vi "Camera_Crop_Setup.vi"(11 "value":T1={"L16 Linear Actuator"="", "XE 1000 Pump"="", "Camera1"="", "Camera2"="", "Img_Capt"=FALSE, "Actuator"=FALSE, "Pump"=FALSE, "Cam 1"=FALSE, "Cam 2"=FALSE, "Empty_Refill"=FALSE, "Crop"=FALSE, "Light intensity"=100, "Exposure Time"=1000.0, "Sample Name"="Test Sample", "Operator"="MRJ", "Calibration 1"=path "C:/Users/au540322/Desktop/IHS_Project/images/Debris/Debris_0/Debris_0_2019_06_01-23-32-49-686.PNG", "Calibration 2"=path "C:/Users/au540322/Desktop/IHS_Project/images/Debris/Debris_0/Debris_0_2019_06_01-23-32-49-686.PNG", "Framerate"=100, "Timeout Sample"=200, "Collection date"="", "Sample size threshold"=500, "Empty start"=1, "Command"="", "Station"="", "Species Name"="", "Other Notes"="", "Aperture"=enum."Item 0", "Image Process Queue Size"=500, "Image Save Queue Size"=500, "Overload threshold"=500, "Max Framerate"=100, "Rectangle 1"={"Left"=0, "Top"=0, "Right"=0, "Bottom"=0, "Rotation"=0.0}, "Rectangle 2"={"Left"=0, "Top"=0, "Right"=0, "Bottom"=0, "Rotation"=0.0}, "Detection Region %"=0.0, "Detect 1"=path "C:/Users/au540322/Desktop/IHS_Project/images/Debris/Debris_0/Debris_0_2019_06_01-23-32-49-686.PNG", "Detect 2"=path "C:/Users/au540322/Desktop/IHS_Project/images/Debris/Debris_0/Debris_0_2019_06_01-23-32-49-686.PNG", "Max large object threshold"=0, "Open(T)/Close(F)"=FALSE, "Img_Capt Begin"=FALSE, "Dispense Speed"=100, "Flush Size"=100, "Location"="Station", "Latitude"="Station", "Longitude"="Station", "Determiner"="Station", "Sex"="Station", "Camera1_Img"=refnum, "Camera2_Img"=refnum, "Img1_Orig_Disp"=refnum, "Img2_Orig_Disp"=refnum, "Img1_Orig_RGB"=refnum, "Img2_Orig_RGB"=refnum, "Blue_Plane_Extract"=refnum, "Subtracted_Plane"=refnum, "Img1_Binary"=refnum, "Img2_Binary"=refnum, "Crop_Mask"=refnum, "Img1_Save"=refnum, "Img2_Save"=refnum, "Img1_Cali_Full"=refnum, "Img2_Cali_Full"=refnum, "Img1_Cali_Detect"=refnum, "Img2_Cali_Detect"=refnum, "Cam 1 queue"=refnum, "Cam 2 queue"=refnum, "Cam 1 - save queue"=refnum, "Cam 2 - save queue"=refnum, "Overlay_Ring"=0, "SystemVersion"=0, "System Serial"=""} {"SystemVersion" items=["Standard", "XL"]; "Overlay_Ring" items=["Session Data", "Extended Setup", "Buffer", "Camera", "Dispenser", "Stats", "Connections"]; "Flush Size" min=1; "Dispense Speed" min=1; "Rectangle 2"."Rotation" format="%.2f"; "Rectangle 2"."Left" scale=0.0..1024.0; "Rectangle 2"."Right" scale=0.0..1024.0; "Rectangle 1"."Rotation" format="%.2f"; "Rectangle 1"."Left" scale=0.0..1024.0; "Rectangle 1"."Right" scale=0.0..1024.0; "Max Framerate" min=1; "Overload threshold" min=1; "Image Save Queue Size" min=1; "Image Process Queue Size" min=1; "Empty start" min=1; "Sample size threshold" min=1; "Framerate" min=1; "Light intensity" scale=0.0..100.0}) -> (3 "output cluster":T1={"L16 Linear Actuator"="", "XE 1000 Pump"="", "Camera1"="", "Camera2"="", "Img_Capt"=FALSE, "Actuator"=FALSE, "Pump"=FALSE, "Cam 1"=FALSE, "Cam 2"=FALSE, "Empty_Refill"=FALSE, "Crop"=FALSE, "Light intensity"=100, "Exposure Time"=1000.0, "Sample Name"="Test Sample", "Operator"="MRJ", "Calibration 1"=path "C:/Users/au540322/Desktop/IHS_Project/images/Debris/Debris_0/Debris_0_2019_06_01-23-32-49-686.PNG", "Calibration 2"=path "C:/Users/au540322/Desktop/IHS_Project/images/Debris/Debris_0/Debris_0_2019_06_01-23-32-49-686.PNG", "Framerate"=100, "Timeout Sample"=200, "Collection date"="", "Sample size threshold"=500, "Empty start"=1, "Command"="", "Station"="", "Species Name"="", "Other Notes"="", "Aperture"=enum."Item 0", "Image Process Queue Size"=500, "Image Save Queue Size"=500, "Overload threshold"=500, "Max Framerate"=100, "Rectangle 1"={"Left"=0, "Top"=0, "Right"=0, "Bottom"=0, "Rotation"=0.0}, "Rectangle 2"={"Left"=0, "Top"=0, "Right"=0, "Bottom"=0, "Rotation"=0.0}, "Detection Region %"=0.0, "Detect 1"=path "C:/Users/au540322/Desktop/IHS_Project/images/Debris/Debris_0/Debris_0_2019_06_01-23-32-49-686.PNG", "Detect 2"=path "C:/Users/au540322/Desktop/IHS_Project/images/Debris/Debris_0/Debris_0_2019_06_01-23-32-49-686.PNG", "Max large object threshold"=0, "Open(T)/Close(F)"=FALSE, "Img_Capt Begin"=FALSE, "Dispense Speed"=100, "Flush Size"=100, "Location"="Station", "Latitude"="Station", "Longitude"="Station", "Determiner"="Station", "Sex"="Station", "Camera1_Img"=refnum, "Camera2_Img"=refnum, "Img1_Orig_Disp"=refnum, "Img2_Orig_Disp"=refnum, "Img1_Orig_RGB"=refnum, "Img2_Orig_RGB"=refnum, "Blue_Plane_Extract"=refnum, "Subtracted_Plane"=refnum, "Img1_Binary"=refnum, "Img2_Binary"=refnum, "Crop_Mask"=refnum, "Img1_Save"=refnum, "Img2_Save"=refnum, "Img1_Cali_Full"=refnum, "Img2_Cali_Full"=refnum, "Img1_Cali_Detect"=refnum, "Img2_Cali_Detect"=refnum, "Cam 1 queue"=refnum, "Cam 2 queue"=refnum, "Cam 1 - save queue"=refnum, "Cam 2 - save queue"=refnum, "Overlay_Ring"=0, "SystemVersion"=0, "System Serial"=""} {"SystemVersion" items=["Standard", "XL"]; "Overlay_Ring" items=["Session Data", "Extended Setup", "Buffer", "Camera", "Dispenser", "Stats", "Connections"]; "Flush Size" min=1; "Dispense Speed" min=1; "Rectangle 2"."Rotation" format="%.2f"; "Rectangle 2"."Left" scale=0.0..1024.0; "Rectangle 2"."Right" scale=0.0..1024.0; "Rectangle 1"."Rotation" format="%.2f"; "Rectangle 1"."Left" scale=0.0..1024.0; "Rectangle 1"."Right" scale=0.0..1024.0; "Max Framerate" min=1; "Overload threshold" min=1; "Image Save Queue Size" min=1; "Image Process Queue Size" min=1; "Empty start" min=1; "Sample size threshold" min=1; "Framerate" min=1; "Light intensity" scale=0.0..100.0})   [LabVIEW 2021]
uses:
  controls/Data.ctl
  <vilib>/userDefined/High Color/IMAQdx.ctl
  <vilib>/vision/Image Controls.llb/IMAQ Image.ctl
types:
  T1 = typedef "Data.ctl" = cluster{"L16 Linear Actuator":refnum<visa-resource-name>, "XE 1000 Pump":refnum<visa-resource-name>, "Camera1":T2, "Camera2":T2, "Img_Capt":bool, "Actuator":bool, "Pump":bool, "Cam 1":bool, "Cam 2":bool, "Empty_Refill":bool, "Crop":bool, "Light intensity":i32, "Exposure Time":dbl, "Sample Name":string, "Operator":string, "Calibration 1":path, "Calibration 2":path, "Framerate":i32, "Timeout Sample":i32, "Collection date":string, "Sample size threshold":i32, "Empty start":u32, "Command":string, "Station":string, "Species Name":string, "Other Notes":string, "Aperture":enum32{"Item 0", "Item 1", "Item 2", "Item 3"}, "Image Process Queue Size":i32, "Image Save Queue Size":i32, "Overload threshold":i32, "Max Framerate":i32, "Rectangle 1":T3, "Rectangle 2":T3, "Detection Region %":dbl, "Detect 1":path, "Detect 2":path, "Max large object threshold":i32, "Open(T)/Close(F)":bool, "Img_Capt Begin":bool, "Dispense Speed":i32, "Flush Size":i32, "Location":string, "Latitude":string, "Longitude":string, "Determiner":string, "Sex":string, "Camera1_Img":T4, "Camera2_Img":T4, "Img1_Orig_Disp":T4, "Img2_Orig_Disp":T4, "Img1_Orig_RGB":T4, "Img2_Orig_RGB":T4, "Blue_Plane_Extract":T4, "Subtracted_Plane":T4, "Img1_Binary":T4, "Img2_Binary":T4, "Crop_Mask":T4, "Img1_Save":T4, "Img2_Save":T4, "Img1_Cali_Full":T4, "Img2_Cali_Full":T4, "Img1_Cali_Detect":T4, "Img2_Cali_Detect":T4, "Cam 1 queue":refnum<queue>, "Cam 2 queue":refnum<queue>, "Cam 1 - save queue":refnum<queue>, "Cam 2 - save queue":refnum<queue>, "Overlay_Ring":u16, "SystemVersion":u16, "System Serial":string}
  T2 = typedef "IMAQdx.ctl" = refnum<k21>
  T3 = typedef "IMAQ Rectangle" = cluster{"Left":i32, "Top":i32, "Right":i32, "Bottom":i32, "Rotation":dbl}
  T4 = typedef "IMAQ Image.ctl" = refnum<image>
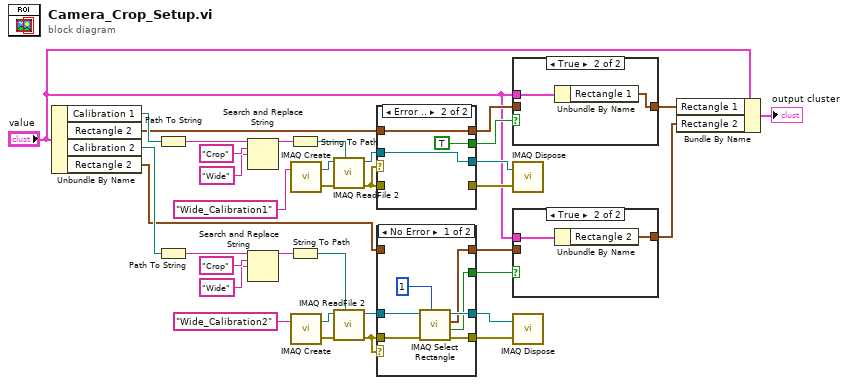
[diagram p0: block diagram]
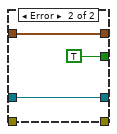
[diagram p4: hidden frame]
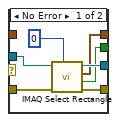
[diagram p5: hidden frame]
diagram:
  n1 = Unbundle By Name("value") -> ("Calibration 1"=w10:path, "Rectangle 2"=w9:T3, "Calibration 2"=w12:path, "Rectangle 2"=w11:T3)
  n2 = Path To String(path=w10) -> (string=w32:string)
  n3 = Path To String(path=w12) -> (string=w20:string)
  n4 = Search and Replace String(input string=w32, search string="Crop", replace string="Wide" ("replace string (\"\")")) -> (result string=w29:string)  [unwired: 5 in, 3 out]
  n5 = Search and Replace String(input string=w20, search string="Crop", replace string="Wide" ("replace string (\"\")")) -> (result string=w17:string)  [unwired: 5 in, 3 out]
  n6 = String To Path(string=w29) -> (path=w28:path)
  n7 = String To Path(string=w17) -> (path=w16:path)
  n8 = call "IMAQ Create"("Image Name"="Wide_Calibration1") -> ("New Image"=w36:T4, "error out"=w33:errorcluster)  [unwired: 4 in]
  n9 = call "IMAQ Create"("Image Name"="Wide_Calibration2") -> ("New Image"=w24:T4, "error out"=w21:errorcluster)  [unwired: 4 in]
  n10 = call "IMAQ ReadFile 2"("File Path"=w28, "error in (no error)"=w33, "Image"=w36) -> ("error out"=w27:errorcluster, "Image Out"=w34:T4)  [unwired: 4 in, 3 out]
  n11 = call "IMAQ ReadFile 2"("File Path"=w16, "error in (no error)"=w21, "Image"=w24) -> ("error out"=w15:errorcluster, "Image Out"=w22:T4)  [unwired: 4 in, 3 out]
  n12 = case shown="Error .." w27 {
    tunnel: w34 -> [w43 w46]
    tunnel: w27 -> [w42 _]
    tunnel: [w40 w46] -> w26
    tunnel: [w39 _] -> w25
    tunnel: [w38 w45] -> w6
    tunnel: w9 -> [_ w45]
    tunnel: [w37 TRUE ("Cancelled")] -> w8
    frame No Error {
      n13 = call "IMAQ Select Rectangle"("Window Number (0...15)"=0, "error in (no error)"=w42, "Image In"=w43) -> ("error out"=w39:errorcluster, "Cancelled"=w37:bool, "Rectangle"=w38:T3, "Image Out (duplicate)"=w40:T4)  [unwired: 5 in]
    }
    frame Error {
    }
  }
  n14 = case shown="No Error" w15 {
    tunnel: w22 -> [w53 w56]
    tunnel: w15 -> [w52 _]
    tunnel: [w50 w56] -> w14
    tunnel: [w49 _] -> w13
    tunnel: [w48 w55] -> w3
    tunnel: w11 -> [_ w55]
    tunnel: [w47 TRUE ("Cancelled")] -> w5
    frame No Error {
      n15 = call "IMAQ Select Rectangle"("Window Number (0...15)"=1, "error in (no error)"=w52, "Image In"=w53) -> ("error out"=w49:errorcluster, "Cancelled"=w47:bool, "Rectangle"=w48:T3, "Image Out (duplicate)"=w50:T4)  [unwired: 5 in]
    }
    frame Error {
    }
  }
  n16 = case shown="True" w8 {
    tunnel: [w57 w59] -> w7
    tunnel: w6 -> [w57 _]
    tunnel: "value" -> [_ w58]
    frame False {
    }
    frame True {
      n17 = Unbundle By Name(w58) -> ("Rectangle 1"=w59:T3)
    }
  }
  n18 = call "IMAQ Dispose"("Image"=w26, "error in (no error)"=w25) -> ()  [unwired: 4 in, 1 out]
  n19 = case shown="True" w5 {
    tunnel: "value" -> [_ w62]
    tunnel: w3 -> [w60 _]
    tunnel: [w60 w61] -> w4
    frame False {
    }
    frame True {
      n20 = Unbundle By Name(w62) -> ("Rectangle 2"=w61:T3)
    }
  }
  n21 = call "IMAQ Dispose"("Image"=w14, "error in (no error)"=w13) -> ()  [unwired: 4 in, 1 out]
  n22 = Bundle By Name(cluster="value", "Rectangle 1"=w7, "Rectangle 2"=w4) -> (→"output cluster":T1)
